vi "CHS_Robot Main.vi"() -> ()   [LabVIEW 2019]
doc: "This VI implements the framework and scheduler for your robotics program. It should not be necessary to modify the framework. You are expected to add your code to the VIs called from Robot Main - the ones located in the Team Code folder within the project."
uses:
  <vilib>/Rock Robotics/WPI/Camera/WPI_CameraImageSize.ctl
  SubVI/CHS_Robot Global Data.vi
  <vilib>/Rock Robotics/WPI/ThirdParty/JAS_Junk/TrajLib/Trajectory_Library.lvlib
panel:
  in  "DisplayField":string(combo)
  in  "Image Size":T1=enum."320x240"
  in  "Enable Vision":bool
  in  "Finish":bool
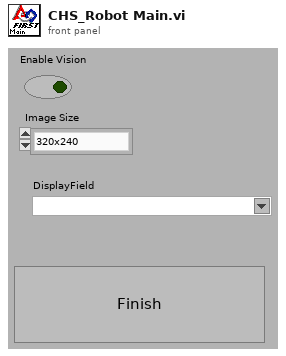
[diagram p1: front panel]
types:
  T1 = typedef "WPI_CameraImageSize.ctl" = enum16{"640x480", "320x240", "160x120", "Custom"}
  T2 = enum32{"Invalid", "Standard", "Closed", "Hidden", "Minimized", "Maximized"}
  T3 = typedef "WPI_DriverStationMatch Info.ctl" = cluster{"Autonomous Elapsed Seconds":dbl, "TeleOp Elapsed Seconds":dbl, "Disabled Elapsed Seconds":dbl, "Visited Autonomous":bool, "Visited TeleOp":bool, "Visited Disabled":bool, "Autonomous Settings":cluster{"Autonomous Style":enum16{"Iterative", "Independent"}, "VI Refnum":refnum<vi>}}
  T4 = typedef "WPI_DriverStationDerivedRobotMode.ctl" = enum16{"Init", "Execute", "Stop"}
  T5 = typedef "WPI_DriverStationRobotMode2.ctl" = enum16{"Autonomous Disabled", "Autonomous Enabled", "Teleop Disabled", "Teleop Enabled", "Disconnected", "Finish", "Test Disabled", "Test Enabled", "Emergency Stopped"}
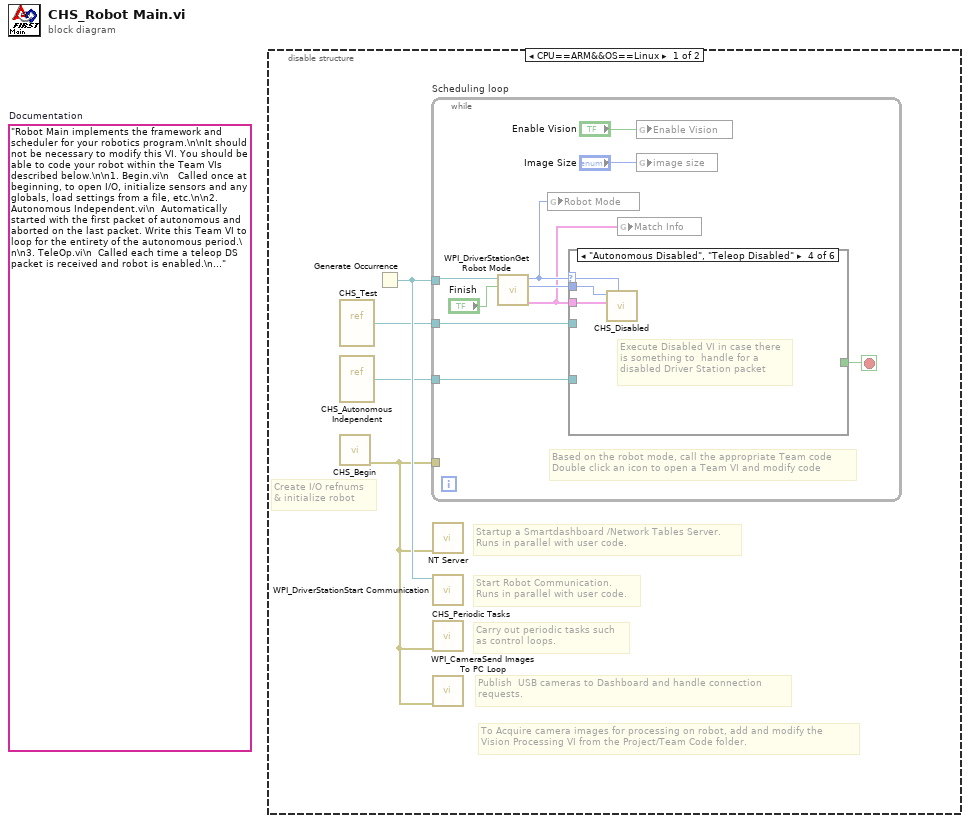
[diagram p0: block diagram]
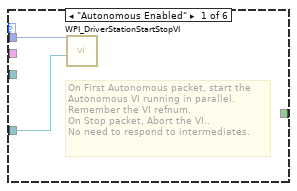
[diagram p2: hidden frame]
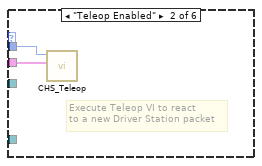
[diagram p3: hidden frame]
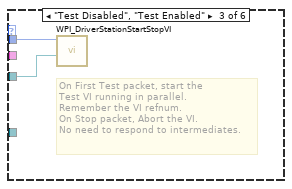
[diagram p4: hidden frame]
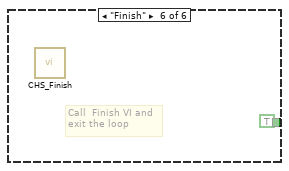
[diagram p6: hidden frame]
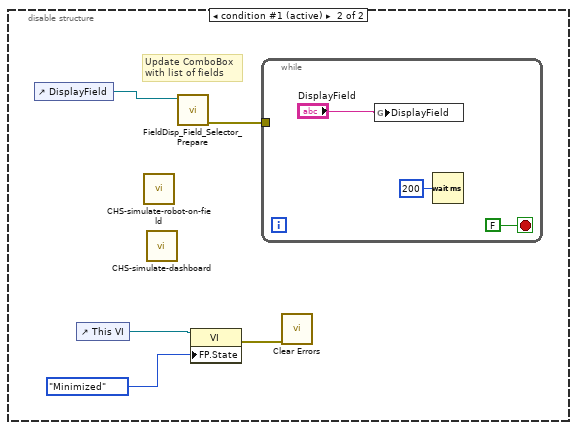
[diagram p7: hidden frame]
diagram:
  (unwired) "Robot Main implements the framework and scheduler for your robotics program.\n\nIt should not be necessary to modify this VI. You should be able to code your robot within the Team VIs described below.\n\n1. Begin.vi\n   Called once at beginning, to open I/O, initialize sensors and any globals, load settings from a file, etc.\n\n2. Autonomous Independent.vi\n  Automatically started with the first packet of autonomous and aborted on the last packet. Write this Team VI to loop for the entirety of the autonomous period.\n\n3. TeleOp.vi\n  Called each time a teleop DS packet is received and robot is enabled.\n\n4. Disabled.vi\n  Called each time a packet is received and the robot is disabled.\n\n5. Test.vi\n  Called Automatically started with the first test packet and aborted on the last. Modify this VI to carry out robot and sensor validation tests.\n\n6. Vision Processing.vi\n  A parallel loop that acquires and processes camera images. Drag from the project/Team Code if you wish to use this.\n\n7. PeriodicTasks.vi\n  Parallel loops running at user-defined rates.\n\n8. Finish.vi\n  Called before exiting, so you can save data, clean up I/O, etc.\n"  # Documentation
  n1 = disable-structure shown="CPU==ARM&&OS==Linux" {
    frame condition #0 {
      # "Publish  USB cameras to Dashboard and handle connection\nrequests."
      # "Startup a Smartdashboard /Network Tables Server.\nRuns in parallel with user code."
      # "Carry out periodic tasks such\nas control loops."
      # "To Acquire camera images for processing on robot, add and modify the\nVision Processing VI from the Project/Team Code folder."
      # "Create I/O refnums\n& initialize robot"
      # "Start Robot Communication.\nRuns in parallel with user code."
      n2 = vi-ref "CHS_Test.vi"() -> (w2:refnum<vi>)
      n3 = vi-ref "CHS_Autonomous Independent.vi"() -> (w3:refnum<vi>)
      n4 = call "CHS_Begin.vi"() -> ("error out"=w1:errorcluster)  [unwired: 2 in, 9 out]
      n5 = Generate Occurrence() -> (w4:refnum<k4>)
      n6 = while "Scheduling loop" {
        tunnel: w4 -> [w13]
        tunnel: w1 -> [_]
        tunnel: w3 -> [w9]
        tunnel: w2 -> [w7]
        stop <- w11 stop-if-true
        # "Based on the robot mode, call the appropriate Team code\nDouble click an icon to open a Team VI and modify code"
        n7 = call <vilib>:"WPI_DriverStationGet Robot Mode.vi"("Finish"="Finish", "DS Occurrence"=w13) -> ("Match Info out"=w5:T3, "Call Context"=w14:T4, "Robot Mode"=w6:T5)  [unwired: 7 out]
        n8 = global write "CHS_Robot Global Data.vi" "Robot Mode"(w6) -> ()
        n9 = case shown="\"Autonomous Disabled\", \"Teleop Disabled\"" w6 {
          selector: w6 -> [_ _ _ w21 _ _]
          tunnel: w14 -> [w16 w18 w20 w23 _ _]
          tunnel: w5 -> [_ w17 _ w22 _ _]
          tunnel: [_ _ _ _ _ TRUE] -> w11
          tunnel: w9 -> [w15 _ _ _ _ _]
          tunnel: w7 -> [_ _ w19 _ _ _]
          frame "Autonomous Enabled" {
            # "On First Autonomous packet, start the\nAutonomous VI running in parallel.\nRemember the VI refnum.\nOn Stop packet, Abort the VI..\nNo need to respond to intermediates."
            n10 = call <vilib>:"WPI_DriverStationStartStopVI.vi"("VI in"=w15, "Call Context"=w16) -> ()  [unwired: 10 in]
          }
          frame "Teleop Enabled" {
            # "Execute Teleop VI to react\nto a new Driver Station packet"
            n11 = call "CHS_Teleop.vi"("Match Info"=w17, "Call Context"=w18) -> ()  [unwired: 1 in, 9 out]
          }
          frame "Test Disabled", "Test Enabled" {
            # "On First Test packet, start the\nTest VI running in parallel.\nRemember the VI refnum.\nOn Stop packet, Abort the VI.\nNo need to respond to intermediates."
            n12 = call <vilib>:"WPI_DriverStationStartStopVI.vi"("VI in"=w19, "Call Context"=w20) -> ()  [unwired: 10 in]
          }
          frame "Autonomous Disabled", "Teleop Disabled" {
            # "Execute Disabled VI in case there\nis something to  handle for a\ndisabled Driver Station packet"
            n13 = call "CHS_Disabled.vi"("Robot Mode"=w21, "Match Info"=w22, "Call Context"=w23) -> ()  [unwired: 1 in, 8 out]
          }
          frame "Disconnected", Default {
            # "Driver Station packet didn't arrive.\nPossibly useful for diagnostics"
          }
          frame "Finish" {
            # "Call  Finish VI and\nexit the loop"
            n14 = call "CHS_Finish.vi"() -> ()  [unwired: 1 in, 7 out]
          }
        }
        n15 = global write "CHS_Robot Global Data.vi" "Match Info"(w5) -> ()
        n16 = global write "CHS_Robot Global Data.vi" "Enable Vision"("Enable Vision") -> ()
        n17 = global write "CHS_Robot Global Data.vi" "image size"("Image Size") -> ()
      }
      n18 = call <vilib>:"NT Server.vi"("error in (no error)"=w1) -> ()  [unwired: 10 in, 1 out]
      n19 = call <vilib>:"WPI_DriverStationStart Communication.vi"("occurrence"=w4) -> ()  [unwired: 2 in, 9 out]
      n20 = call "CHS_Periodic Tasks.vi"("error in"=w1) -> ()  [unwired: 1 in, 10 out]
      n21 = call <vilib>:"WPI_CameraSend Images To PC Loop.vi"("error in (no error)"=w1) -> ()  [unwired: 11 in]
    }
    frame condition #1 (active) {
      # "Update ComboBox\nwith list of fields"
      n22 = control-ref of="DisplayField"() -> (w26:refnum<vi>)
      n23 = control-ref of="This VI"() -> (w29:refnum<vi>)
      n24 = call "CHS-simulate-robot-on-field.vi"() -> ()  [unwired: 12 in]
      n25 = call "CHS-simulate-dashboard.vi"() -> ()  [unwired: 12 in]
      n26 = call <vilib>:"FieldDisp_Field_Selector_Prepare.vi"("ComboBox Ref"=w26) -> ("error out"=w25:errorcluster)  [unwired: 9 in, 1 out]
      n27 = property class="VI"(reference=w29, "FP.State"=T2."Minimized" ("Front Panel Window:State")) -> (error out=w27:errorcluster)  [unwired: 1 in, 1 out]
      n28 = while {
        tunnel: w25 -> [_]
        stop <- FALSE stop-if-true
        n29 = global write "CHS_Robot Global Data.vi" "DisplayField"("DisplayField") -> ()
        n30 = Wait (ms)(milliseconds to wait=u32 200) -> ()  [unwired: 1 out]
      }
      n31 = call <vilib>:"Clear Errors.vi"("error in (no error)"=w27) -> ()  [unwired: 5 in, 2 out]
    }
  }
